vi "Asylum Acquired Data.vi"() -> ()   [LabVIEW 2016]
uses:
  <vilib>/Platform/TimedLoop/XDataNode/timing_clust.ctl
  <vilib>/Platform/TimedLoop/XDataNode/nitl_modes.ctl
  <vilib>/Platform/TimedLoop/XDataNode/wakeup.ctl
  <vilib>/DAQmx/read.llb/DAQmx Read (Analog 1D DBL NChan 1Samp).vi
  subVIs/Driver Variables.vi
  <vilib>/DAQmx/create/channels.llb/DAQmx Create Channel (AI-Voltage-Basic).vi
  <vilib>/DAQmx/configure/timing.llb/DAQmx Timing (Sample Clock).vi
  <vilib>/DAQmx/miscellaneous.llb/DAQmx Fill In Error Info.vi
  <vilib>/Platform/TimedLoop/XDataNode/XDataNode.xnode
  <vilib>/Platform/TimedLoop/XDataNode/XDNodeRunTimeDep.lvlib
panel:
  in  "Reset Graphs":bool
  in  "Data Queue":refnum<queue>
  in  "Skip Back Button":bool
  in  "FF Speed":dbl=2.0
  in  "Progress":dbl(slide)=0.002 scale=0.0..1435.0
  in  "Seek Forward Button":bool
  in  "Media Stop Button":bool
  in  "Play Button":bool
  in  "Tabs":T1(tab)
  in  "Lockin Information":T2={"SR7265 Sensitivity (A)"=5e-07, "Excitation Voltage (V)"=0.1, "SR810 Sensitivity (A)"=0.1, "Femto Gain (V/A)"=1.0, "Frequency (Hz)"=27.0}
  in  "Channel 1 (z, x, y, defl, Vtip, 4t I, 4t V)":tag="Dev1/ai0:3"
  in  "TDMS File Name":string="SA02821"
  in  "TDMS Output Folder":path=path "P:/users1/Yuhe/cypher tdms"
  out "TDMS Path Result":path=path "P:/users1/Yuhe/cypher tdms/SA02821.000109.tdms"
  in  "View Data After?":bool
  out "Z Value":cluster{"Y":dbl[], "Y":dbl[]}[](graph)=[{"Y"=[5.660999774932861, 5.861000061035156, 6.060999870300293, 6.261000156402588, 6.460999965667725, 6.660999774932861, 6.861000061035156, 7.060999870300293, 7.261000156402588, 7.460999965667725, 7.660999774932861, 7.861000061035156, 8.060999870300293, 8.261000156402588, 8.460999965667725, 8.660999774932861, 8.861000061035156, 9.060999870300293, 9.261000156402588, 9.460999965667725, 9.660999774932861, 9.861000061035156, 10.060999870300293, 10.261000156402588, 10.460999965667725, 10.660999774932861, 10.861000061035156, 11.060999870300293, 11.261000156402588, 11.460999965667725, 11.664999961853027, 11.861000061035156, 12.060999870300293, 12.261000156402588, 12.460999965667725, 12.660999774932861, 12.861000061035156, 13.060999870300293, 13.261000156402588, 13.460999965667725, 13.660999774932861, 13.861000061035156, 14.060999870300293, 14.261000156402588, 14.460999965667725, 14.660999774932861, 14.861000061035156, 15.060999870300293, 15.261000156402588, 15.460999965667725, 15.660999774932861, 15.861000061035156, 16.060999870300293, 16.261000156402588, 16.460999965667725, 16.65999984741211, 16.860000133514404, 17.05999994277954, 17.260000228881836, 17.460000038146973, 17.65999984741211, 17.860000133514404, 18.05999994277954, 18.260000228881836, 18.460000038146973, 18.65999984741211, 18.860000133514404, 19.05999994277954, 19.260000228881836, 19.460000038146973, 19.65999984741211, 19.860000133514404, 20.05999994277954, 20.260000228881836, 20.460000038146973, 20.65999984741211, 20.860000133514404, 21.05999994277954, 21.260000228881836, 21.460000038146973, 21.65999984741211, 21.860000133514404, 22.05999994277954, 22.260000228881836, 22.460000038146973, 22.65999984741211, 22.86299991607666, 23.05999994277954, 23.260000228881836, 23.460000038146973, 23.65999984741211, 23.860000133514404, 24.05999994277954, 24.260000228881836, 24.461999893188477, 24.65999984741211, 24.860000133514404, 25.05999994277954, 25.260000228881836, 25.460000038146973, 25.65999984741211, 25.860000133514404, 26.05999994277954, 26.260000228881836, 26.460000038146973], "Y"=[-4.029889960155487, -4.029913362326622, -4.030140697703361, -4.029893303322791, -4.0299033328247065, -4.029686026949883, -4.029659281611442, -4.029562329759599, -4.029849842147827, -4.028997334485054, -4.029719458622933, -4.029826439976692, -4.029873244318962, -4.029833126311303, -4.0292781605386745, -4.029712772288322, -4.029849842147827, -4.029976882505417, -4.0298230968093876, -4.0300303731822975, -4.029535584421158, -4.029806380972862, -4.029916705493927, -4.029910019159317, -4.028963902812004, -4.029986912007331, -4.029776292467117, -4.029923391828537, -4.029960166668892, -4.0288268329524985, -4.030164099874496, -4.029866557984352, -4.030020343680382, -4.029853185315133, -4.029719458622933, -4.029712772288322, -4.029742860794068, -4.029692713284493, -4.030067148022652, -4.029077570500373, -4.030050432186126, -4.029896646490098, -4.029970196170807, -4.029916705493927, -4.029167836017609, -4.029866557984352, -4.0296425657749175, -4.029839812645912, -4.029652595276832, -4.029956823501586, -4.029722801790237, -4.029943450832366, -4.029913362326622, -4.029873244318962, -4.029030766158105, -4.029893303322791, -4.0297328312921525, -4.029809724140167, -4.029502152748108, -4.0292781605386745, -4.029849842147827, -4.0298632148170475, -4.030134011368751, -4.029829783143997, -4.0288268329524985, -4.029776292467117, -4.029933421330452, -4.029525554919243, -4.0298230968093876, -4.0287867149448395, -4.029846498980523, -4.0294754074096675, -4.0296693111133575, -4.029652595276832, -4.028890353131294, -4.029762919797897, -4.029645908942223, -4.029866557984352, -4.029889960155487, -4.028582781739235, -4.029585731930733, -4.029776292467117, -4.029689370117188, -4.029826439976692, -4.029953480334282, -4.029696056451798, -4.030077177524567, -4.029809724140167, -4.0295656729269025, -4.0288769804620745, -4.0299668530035015, -4.029803037805558, -4.030190845212937, -4.029652595276832, -4.030087207026482, -4.029769606132508, -4.029635879440308, -4.029813067307472, -4.029910019159317, -4.029094286336899, -4.0297328312921525, -4.029488780078888, -4.029956823501586, -4.029853185315133, -4.029087600002288]}]
  out "X Position":cluster{"Y":dbl[], "Y":dbl[]}[](graph)=[{"Y"=[5.660999774932861, 5.861000061035156, 6.060999870300293, 6.261000156402588, 6.460999965667725, 6.660999774932861, 6.861000061035156, 7.060999870300293, 7.261000156402588, 7.460999965667725, 7.660999774932861, 7.861000061035156, 8.060999870300293, 8.261000156402588, 8.460999965667725, 8.660999774932861, 8.861000061035156, 9.060999870300293, 9.261000156402588, 9.460999965667725, 9.660999774932861, 9.861000061035156, 10.060999870300293, 10.261000156402588, 10.460999965667725, 10.660999774932861, 10.861000061035156, 11.060999870300293, 11.261000156402588, 11.460999965667725, 11.664999961853027, 11.861000061035156, 12.060999870300293, 12.261000156402588, 12.460999965667725, 12.660999774932861, 12.861000061035156, 13.060999870300293, 13.261000156402588, 13.460999965667725, 13.660999774932861, 13.861000061035156, 14.060999870300293, 14.261000156402588, 14.460999965667725, 14.660999774932861, 14.861000061035156, 15.060999870300293, 15.261000156402588, 15.460999965667725, 15.660999774932861, 15.861000061035156, 16.060999870300293, 16.261000156402588, 16.460999965667725, 16.65999984741211, 16.860000133514404, 17.05999994277954, 17.260000228881836, 17.460000038146973, 17.65999984741211, 17.860000133514404, 18.05999994277954, 18.260000228881836, 18.460000038146973, 18.65999984741211, 18.860000133514404, 19.05999994277954, 19.260000228881836, 19.460000038146973, 19.65999984741211, 19.860000133514404, 20.05999994277954, 20.260000228881836, 20.460000038146973, 20.65999984741211, 20.860000133514404, 21.05999994277954, 21.260000228881836, 21.460000038146973, 21.65999984741211, 21.860000133514404, 22.05999994277954, 22.260000228881836, 22.460000038146973, 22.65999984741211, 22.86299991607666, 23.05999994277954, 23.260000228881836, 23.460000038146973, 23.65999984741211, 23.860000133514404, 24.05999994277954, 24.260000228881836, 24.461999893188477, 24.65999984741211, 24.860000133514404, 25.05999994277954, 25.260000228881836, 25.460000038146973, 25.65999984741211, 25.860000133514404, 26.05999994277954, 26.260000228881836, 26.460000038146973], "Y"=[4.567807958678547, 4.578632321776692, 4.575999827613178, 4.570083792342488, 4.572387932395284, 4.567892877845113, 4.5784454996102495, 4.576243262557331, 4.568481650733296, 4.572693641394917, 4.567853248900715, 4.578802160109822, 4.577307582778279, 4.567428653067891, 4.572982366561238, 4.566811573790853, 4.578666289443317, 4.575846973113362, 4.568175941733663, 4.573129559783284, 4.568815666121785, 4.576679180945699, 4.576107391890828, 4.57247851283962, 4.572659673728292, 4.568532602233234, 4.578541741332355, 4.576724471167866, 4.570383840064351, 4.572263384284321, 4.566709670790974, 4.577443453444783, 4.576639552001301, 4.5702026791756785, 4.572925753783528, 4.567151250457113, 4.578371902999226, 4.577109438056294, 4.572778560561482, 4.573180511283223, 4.569381793898884, 4.5792154333871045, 4.576826374167744, 4.570389501342122, 4.573180511283223, 4.568685456733052, 4.578405870665852, 4.576752777556721, 4.571125467452352, 4.573288075560871, 4.5689005852883495, 4.579113530387227, 4.577183034667317, 4.568487312011068, 4.57270496395046, 4.570916000174824, 4.578932369498554, 4.576464052390401, 4.568651489066426, 4.573214478949848, 4.568742069510762, 4.578654966887775, 4.576849019278828, 4.570797113341634, 4.572552109450641, 4.569495019454305, 4.579034272498433, 4.574612814559284, 4.567281459845845, 4.572801205672566, 4.568793021010701, 4.579124852942769, 4.5765999230569046, 4.5686118601220285, 4.573248446616474, 4.568532602233234, 4.579577755164448, 4.577109438056294, 4.568991165732686, 4.57276723800594, 4.5694440679543655, 4.579441884497944, 4.57680372905666, 4.572059578284565, 4.5720765621178785, 4.569223278121296, 4.575014765281026, 4.576265907668415, 4.567049347457234, 4.572738931617085, 4.565662334403339, 4.579209772109333, 4.577013196334187, 4.574312766837422, 4.572427561339681, 4.569987550620381, 4.578892740554157, 4.5765716166680495, 4.569149681510274, 4.572750254172627, 4.5689062465661205, 4.57850777366573, 4.576135698279683, 4.5765999230569046, 4.572637028617207]}]
  out "Y Position":cluster{"Y":dbl[], "Y":dbl[]}[](graph)=[{"Y"=[5.660999774932861, 5.861000061035156, 6.060999870300293, 6.261000156402588, 6.460999965667725, 6.660999774932861, 6.861000061035156, 7.060999870300293, 7.261000156402588, 7.460999965667725, 7.660999774932861, 7.861000061035156, 8.060999870300293, 8.261000156402588, 8.460999965667725, 8.660999774932861, 8.861000061035156, 9.060999870300293, 9.261000156402588, 9.460999965667725, 9.660999774932861, 9.861000061035156, 10.060999870300293, 10.261000156402588, 10.460999965667725, 10.660999774932861, 10.861000061035156, 11.060999870300293, 11.261000156402588, 11.460999965667725, 11.664999961853027, 11.861000061035156, 12.060999870300293, 12.261000156402588, 12.460999965667725, 12.660999774932861, 12.861000061035156, 13.060999870300293, 13.261000156402588, 13.460999965667725, 13.660999774932861, 13.861000061035156, 14.060999870300293, 14.261000156402588, 14.460999965667725, 14.660999774932861, 14.861000061035156, 15.060999870300293, 15.261000156402588, 15.460999965667725, 15.660999774932861, 15.861000061035156, 16.060999870300293, 16.261000156402588, 16.460999965667725, 16.65999984741211, 16.860000133514404, 17.05999994277954, 17.260000228881836, 17.460000038146973, 17.65999984741211, 17.860000133514404, 18.05999994277954, 18.260000228881836, 18.460000038146973, 18.65999984741211, 18.860000133514404, 19.05999994277954, 19.260000228881836, 19.460000038146973, 19.65999984741211, 19.860000133514404, 20.05999994277954, 20.260000228881836, 20.460000038146973, 20.65999984741211, 20.860000133514404, 21.05999994277954, 21.260000228881836, 21.460000038146973, 21.65999984741211, 21.860000133514404, 22.05999994277954, 22.260000228881836, 22.460000038146973, 22.65999984741211, 22.86299991607666, 23.05999994277954, 23.260000228881836, 23.460000038146973, 23.65999984741211, 23.860000133514404, 24.05999994277954, 24.260000228881836, 24.461999893188477, 24.65999984741211, 24.860000133514404, 25.05999994277954, 25.260000228881836, 25.460000038146973, 25.65999984741211, 25.860000133514404, 26.05999994277954, 26.260000228881836, 26.460000038146973], "Y"=[4.795882738326846, 4.79540291292554, 4.795653730748949, 4.795550132082758, 4.795713708924112, 4.795871833204089, 4.79597543187028, 4.795708256362734, 4.795871833204089, 4.795610110257922, 4.796166271518525, 4.795555584644137, 4.796111745904742, 4.795953621624766, 4.795604657696543, 4.795871833204089, 4.795915453695117, 4.7958118550289255, 4.795708256362734, 4.796068125413713, 4.795642825626193, 4.795631920503434, 4.795582847451029, 4.79593726394063, 4.795839117835818, 4.795997242115793, 4.79554467952138, 4.795740971731005, 4.795959074186144, 4.795708256362734, 4.795795497344789, 4.795501059030352, 4.7962262496936905, 4.79601359979993, 4.796160818957148, 4.795653730748949, 4.796024504922686, 4.795855475519953, 4.795997242115793, 4.795539226960002, 4.795866380642709, 4.795773687099277, 4.795670088433086, 4.7957682345378965, 4.795680993555842, 4.795915453695117, 4.795517416714487, 4.795882738326846, 4.795855475519953, 4.795746424292384, 4.796264417623338, 4.795730066608247, 4.795664635871706, 4.796057220290956, 4.795800949906168, 4.795991789554415, 4.795326577066241, 4.7961008407819845, 4.795392007802781, 4.7956864461172195, 4.795751876853762, 4.795964526747523, 4.796220797132311, 4.7957028038013565, 4.7962262496936905, 4.795882738326846, 4.796035410045442, 4.79589909601098, 4.7961281035888765, 4.795664635871706, 4.7960190523613075, 4.795724614046869, 4.796024504922686, 4.795610110257922, 4.79629713299161, 4.795746424292384, 4.7958118550289255, 4.795877285765467, 4.796073577975092, 4.795670088433086, 4.79589909601098, 4.7961281035888765, 4.795713708924112, 4.796051767729579, 4.79601359979993, 4.795795497344789, 4.795599205135165, 4.795806402467548, 4.795997242115793, 4.795740971731005, 4.7960463151682005, 4.796073577975092, 4.795588300012407, 4.79594271650201, 4.795893643449602, 4.795806402467548, 4.79594271650201, 4.796035410045442, 4.7957682345378965, 4.795833665274438, 4.7962098920095535, 4.7957682345378965, 4.796035410045442, 4.795953621624766, 4.7959699793089]}]
  out "Tip Deflection":cluster{"Y":dbl[], "Y":dbl[]}[](graph)=[{"Y"=[5.660999774932861, 5.861000061035156, 6.060999870300293, 6.261000156402588, 6.460999965667725, 6.660999774932861, 6.861000061035156, 7.060999870300293, 7.261000156402588, 7.460999965667725, 7.660999774932861, 7.861000061035156, 8.060999870300293, 8.261000156402588, 8.460999965667725, 8.660999774932861, 8.861000061035156, 9.060999870300293, 9.261000156402588, 9.460999965667725, 9.660999774932861, 9.861000061035156, 10.060999870300293, 10.261000156402588, 10.460999965667725, 10.660999774932861, 10.861000061035156, 11.060999870300293, 11.261000156402588, 11.460999965667725, 11.664999961853027, 11.861000061035156, 12.060999870300293, 12.261000156402588, 12.460999965667725, 12.660999774932861, 12.861000061035156, 13.060999870300293, 13.261000156402588, 13.460999965667725, 13.660999774932861, 13.861000061035156, 14.060999870300293, 14.261000156402588, 14.460999965667725, 14.660999774932861, 14.861000061035156, 15.060999870300293, 15.261000156402588, 15.460999965667725, 15.660999774932861, 15.861000061035156, 16.060999870300293, 16.261000156402588, 16.460999965667725, 16.65999984741211, 16.860000133514404, 17.05999994277954, 17.260000228881836, 17.460000038146973, 17.65999984741211, 17.860000133514404, 18.05999994277954, 18.260000228881836, 18.460000038146973, 18.65999984741211, 18.860000133514404, 19.05999994277954, 19.260000228881836, 19.460000038146973, 19.65999984741211, 19.860000133514404, 20.05999994277954, 20.260000228881836, 20.460000038146973, 20.65999984741211, 20.860000133514404, 21.05999994277954, 21.260000228881836, 21.460000038146973, 21.65999984741211, 21.860000133514404, 22.05999994277954, 22.260000228881836, 22.460000038146973, 22.65999984741211, 22.86299991607666, 23.05999994277954, 23.260000228881836, 23.460000038146973, 23.65999984741211, 23.860000133514404, 24.05999994277954, 24.260000228881836, 24.461999893188477, 24.65999984741211, 24.860000133514404, 25.05999994277954, 25.260000228881836, 25.460000038146973, 25.65999984741211, 25.860000133514404, 26.05999994277954, 26.260000228881836, 26.460000038146973], "Y"=[2.325611906051636, 2.325635371208191, 2.325648956298828, 2.3255637407302854, 2.3255452156066894, 2.3254772901535032, 2.3255625057220457, 2.3255933809280394, 2.325564975738525, 2.3255476856231687, 2.3256193161010743, 2.325556330680847, 2.325487170219421, 2.325557565689087, 2.325618081092834, 2.3256650114059445, 2.3255736207962037, 2.32559091091156, 2.3255933809280394, 2.325557565689087, 2.3255896759033203, 2.325609436035156, 2.32554274559021, 2.3255921459197997, 2.325582265853882, 2.3255501556396485, 2.325585970878601, 2.325594615936279, 2.3255625057220457, 2.3255748558044433, 2.325567445755005, 2.3255476856231687, 2.325576090812683, 2.325582265853882, 2.3255835008621215, 2.325634136199951, 2.3256193161010743, 2.3255476856231687, 2.325584735870361, 2.325567445755005, 2.3255600357055664, 2.3254772901535032, 2.325599555969238, 2.3255884408950807, 2.325594615936279, 2.325615611076355, 2.3255476856231687, 2.3255056953430175, 2.325584735870361, 2.325571150779724, 2.3255625057220457, 2.325647721290588, 2.3255291604995727, 2.325600790977478, 2.325597085952759, 2.3255538606643675, 2.3254958152770997, 2.325581030845642, 2.325614376068115, 2.325630431175232, 2.3256230211257933, 2.3255143404006957, 2.3254661750793457, 2.325584735870361, 2.3255625057220457, 2.3255341005325314, 2.325551390647888, 2.32554274559021, 2.325603260993957, 2.3255489206314084, 2.32559091091156, 2.325450119972229, 2.3255884408950807, 2.3255835008621215, 2.3255205154418945, 2.325564975738525, 2.3255538606643675, 2.3255686807632445, 2.325537805557251, 2.3256761264801025, 2.3255007553100584, 2.325597085952759, 2.3255872058868405, 2.3256044960021973, 2.325522985458374, 2.3255439805984497, 2.3255588006973267, 2.325556330680847, 2.3255291604995727, 2.3255884408950807, 2.325504460334778, 2.3256254911422727, 2.325584735870361, 2.325489640235901, 2.325582265853882, 2.3255390405654905, 2.325552625656128, 2.3255785608291624, 2.3256366062164306, 2.325620551109314, 2.3256650114059445, 2.32544517993927, 2.325584735870361, 2.3255242204666136, 2.325658836364746]}]
  out "Tip Voltage":cluster{"Y":dbl[], "Y":dbl[]}[](graph)=[{"Y"=[5.660999774932861, 5.861000061035156, 6.060999870300293, 6.261000156402588, 6.460999965667725, 6.660999774932861, 6.861000061035156, 7.060999870300293, 7.261000156402588, 7.460999965667725, 7.660999774932861, 7.861000061035156, 8.060999870300293, 8.261000156402588, 8.460999965667725, 8.660999774932861, 8.861000061035156, 9.060999870300293, 9.261000156402588, 9.460999965667725, 9.660999774932861, 9.861000061035156, 10.060999870300293, 10.261000156402588, 10.460999965667725, 10.660999774932861, 10.861000061035156, 11.060999870300293, 11.261000156402588, 11.460999965667725, 11.664999961853027, 11.861000061035156, 12.060999870300293, 12.261000156402588, 12.460999965667725, 12.660999774932861, 12.861000061035156, 13.060999870300293, 13.261000156402588, 13.460999965667725, 13.660999774932861, 13.861000061035156, 14.060999870300293, 14.261000156402588, 14.460999965667725, 14.660999774932861, 14.861000061035156, 15.060999870300293, 15.261000156402588, 15.460999965667725, 15.660999774932861, 15.861000061035156, 16.060999870300293, 16.261000156402588, 16.460999965667725, 16.65999984741211, 16.860000133514404, 17.05999994277954, 17.260000228881836, 17.460000038146973, 17.65999984741211, 17.860000133514404, 18.05999994277954, 18.260000228881836, 18.460000038146973, 18.65999984741211, 18.860000133514404, 19.05999994277954, 19.260000228881836, 19.460000038146973, 19.65999984741211, 19.860000133514404, 20.05999994277954, 20.260000228881836, 20.460000038146973, 20.65999984741211, 20.860000133514404, 21.05999994277954, 21.260000228881836, 21.460000038146973, 21.65999984741211, 21.860000133514404, 22.05999994277954, 22.260000228881836, 22.460000038146973, 22.65999984741211, 22.86299991607666, 23.05999994277954, 23.260000228881836, 23.460000038146973, 23.65999984741211, 23.860000133514404, 24.05999994277954, 24.260000228881836, 24.461999893188477, 24.65999984741211, 24.860000133514404, 25.05999994277954, 25.260000228881836, 25.460000038146973, 25.65999984741211, 25.860000133514404, 26.05999994277954, 26.260000228881836, 26.460000038146973], "Y"=[0.0, 0.0, 0.0, 0.0, 0.0, 0.0, 0.0, 0.0, 0.0, 0.0, 0.0, 0.0, 0.0, 0.0, 0.0, 0.0, 0.0, 0.0, 0.0, 0.0, 0.0, 0.0, 0.0, 0.0, 0.0, 0.0, 0.0, 0.0, 0.0, 0.0, 0.0, 0.0, 0.0, 0.0, 0.0, 0.0, 0.0, 0.0, 0.0, 0.0, 0.0, 0.0, 0.0, 0.0, 0.0, 0.0, 0.0, 0.0, 0.0, 0.0, 0.0, 0.0, 0.0, 0.0, 0.0, 0.0, 0.0, 0.0, 0.0, 0.0, 0.0, 0.0, 0.0, 0.0, 0.0, 0.0, 0.0, 0.0, 0.0, 0.0, 0.0, 0.0, 0.0, 0.0, 0.0, 0.0, 0.0, 0.0, 0.0, 0.0, 0.0, 0.0, 0.0, 0.0, 0.0, 0.0, 0.0, 0.0, 0.0, 0.0, 0.0, 0.0, 0.0, 0.0, 0.0, 0.0, 0.0, 0.0, 0.0, 0.0, 0.0, 0.0, 0.0, 0.0, 0.0]}]
  out "2-Terminal Conductance":cluster{"Y":dbl[], "Y":dbl[]}[](graph)=[{"Y"=[5.660999774932861, 5.861000061035156, 6.060999870300293, 6.261000156402588, 6.460999965667725, 6.660999774932861, 6.861000061035156, 7.060999870300293, 7.261000156402588, 7.460999965667725, 7.660999774932861, 7.861000061035156, 8.060999870300293, 8.261000156402588, 8.460999965667725, 8.660999774932861, 8.861000061035156, 9.060999870300293, 9.261000156402588, 9.460999965667725, 9.660999774932861, 9.861000061035156, 10.060999870300293, 10.261000156402588, 10.460999965667725, 10.660999774932861, 10.861000061035156, 11.060999870300293, 11.261000156402588, 11.460999965667725, 11.664999961853027, 11.861000061035156, 12.060999870300293, 12.261000156402588, 12.460999965667725, 12.660999774932861, 12.861000061035156, 13.060999870300293, 13.261000156402588, 13.460999965667725, 13.660999774932861, 13.861000061035156, 14.060999870300293, 14.261000156402588, 14.460999965667725, 14.660999774932861, 14.861000061035156, 15.060999870300293, 15.261000156402588, 15.460999965667725, 15.660999774932861, 15.861000061035156, 16.060999870300293, 16.261000156402588, 16.460999965667725, 16.65999984741211, 16.860000133514404, 17.05999994277954, 17.260000228881836, 17.460000038146973, 17.65999984741211, 17.860000133514404, 18.05999994277954, 18.260000228881836, 18.460000038146973, 18.65999984741211, 18.860000133514404, 19.05999994277954, 19.260000228881836, 19.460000038146973, 19.65999984741211, 19.860000133514404, 20.05999994277954, 20.260000228881836, 20.460000038146973, 20.65999984741211, 20.860000133514404, 21.05999994277954, 21.260000228881836, 21.460000038146973, 21.65999984741211, 21.860000133514404, 22.05999994277954, 22.260000228881836, 22.460000038146973, 22.65999984741211, 22.86299991607666, 23.05999994277954, 23.260000228881836, 23.460000038146973, 23.65999984741211, 23.860000133514404, 24.05999994277954, 24.260000228881836, 24.461999893188477, 24.65999984741211, 24.860000133514404, 25.05999994277954, 25.260000228881836, 25.460000038146973, 25.65999984741211, 25.860000133514404, 26.05999994277954, 26.260000228881836, 26.460000038146973], "Y"=[19293.545722961426, 19765.812873840332, 19650.957107543945, 19392.84038543701, 19493.370056152344, 19297.250747680664, 19757.661819458, 19661.57817840576, 19322.938919067383, 19506.708145141598, 19295.52173614502, 19773.22292327881, 19708.014488220215, 19276.996612548828, 19519.30522918701, 19250.073432922363, 19767.294883728027, 19644.288063049316, 19309.600830078125, 19525.72727203369, 19337.512016296387, 19680.597305297848, 19655.65013885498, 19497.32208251953, 19505.226135253906, 19325.161933898926, 19761.86084747314, 19682.573318481445, 19405.93147277832, 19487.93601989746, 19245.627403259277, 19713.942527770996, 19678.868293762203, 19398.027420043945, 19516.83521270752, 19264.893531799316, 19754.450798034664, 19699.369430541992, 19510.41316986084, 19527.950286865234, 19362.212181091305, 19791.2540435791, 19687.01934814453, 19406.17847442627, 19527.950286865234, 19331.830978393555, 19755.932807922367, 19683.80832672119, 19438.288688659668, 19532.64331817627, 19341.21704101562, 19786.80801391602, 19702.580451965332, 19323.185920715332, 19507.2021484375, 19429.149627685547, 19778.903961181644, 19671.21124267578, 19330.34896850586, 19529.43229675293, 19334.300994873047, 19766.800880432125, 19688.007354736324, 19423.96259307861, 19500.53310394287, 19367.152214050293, 19783.349990844727, 19590.441703796387, 19270.57456970215, 19511.401176452637, 19336.52400970459, 19787.30201721191, 19677.139282226562, 19328.619956970215, 19530.914306640625, 19325.161933898926, 19807.062149047848, 19699.369430541992, 19345.169067382812, 19509.91916656494, 19364.92919921875, 19801.13410949707, 19686.031341552734, 19479.04396057129, 19479.784965515133, 19355.29613494873, 19607.97882080078, 19662.566184997555, 19260.44750213623, 19508.68415832519, 19199.93209838867, 19791.007041931152, 19695.170402526855, 19577.350616455078, 19495.09906768799, 19388.641357421875, 19777.174949645996, 19675.904273986816, 19352.08511352539, 19509.178161621094, 19341.464042663574, 19760.37883758545, 19656.885147094727, 19677.139282226562, 19504.23812866211]}]
  out "2-Terminal Resistance":cluster{"Y":dbl[], "Y":dbl[]}[](graph)=[{"Y"=[5.660999774932861, 5.861000061035156, 6.060999870300293, 6.261000156402588, 6.460999965667725, 6.660999774932861, 6.861000061035156, 7.060999870300293, 7.261000156402588, 7.460999965667725, 7.660999774932861, 7.861000061035156, 8.060999870300293, 8.261000156402588, 8.460999965667725, 8.660999774932861, 8.861000061035156, 9.060999870300293, 9.261000156402588, 9.460999965667725, 9.660999774932861, 9.861000061035156, 10.060999870300293, 10.261000156402588, 10.460999965667725, 10.660999774932861, 10.861000061035156, 11.060999870300293, 11.261000156402588, 11.460999965667725, 11.664999961853027, 11.861000061035156, 12.060999870300293, 12.261000156402588, 12.460999965667725, 12.660999774932861, 12.861000061035156, 13.060999870300293, 13.261000156402588, 13.460999965667725, 13.660999774932861, 13.861000061035156, 14.060999870300293, 14.261000156402588, 14.460999965667725, 14.660999774932861, 14.861000061035156, 15.060999870300293, 15.261000156402588, 15.460999965667725, 15.660999774932861, 15.861000061035156, 16.060999870300293, 16.261000156402588, 16.460999965667725, 16.65999984741211, 16.860000133514404, 17.05999994277954, 17.260000228881836, 17.460000038146973, 17.65999984741211, 17.860000133514404, 18.05999994277954, 18.260000228881836, 18.460000038146973, 18.65999984741211, 18.860000133514404, 19.05999994277954, 19.260000228881836, 19.460000038146973, 19.65999984741211, 19.860000133514404, 20.05999994277954, 20.260000228881836, 20.460000038146973, 20.65999984741211, 20.860000133514404, 21.05999994277954, 21.260000228881836, 21.460000038146973, 21.65999984741211, 21.860000133514404, 22.05999994277954, 22.260000228881836, 22.460000038146973, 22.65999984741211, 22.86299991607666, 23.05999994277954, 23.260000228881836, 23.460000038146973, 23.65999984741211, 23.860000133514404, 24.05999994277954, 24.260000228881836, 24.461999893188477, 24.65999984741211, 24.860000133514404, 25.05999994277954, 25.260000228881836, 25.460000038146973, 25.65999984741211, 25.860000133514404, 26.05999994277954, 26.260000228881836, 26.460000038146973], "Y"=[5.1830804682515706e-05, 5.059240449065874e-05, 5.088810659589211e-05, 5.156542209004859e-05, 5.1299492961935945e-05, 5.182085329539442e-05, 5.061327646650814e-05, 5.086061713491017e-05, 5.175196196543506e-05, 5.126441594139825e-05, 5.182549680047088e-05, 5.057344489970375e-05, 5.0740778610535094e-05, 5.1875300914304556e-05, 5.1231331661575256e-05, 5.1947853782716166e-05, 5.058861143530451e-05, 5.090538261251568e-05, 5.178770958549919e-05, 5.121448159486894e-05, 5.1712960755099496e-05, 5.081146595742846e-05, 5.087595642655522e-05, 5.1289094767355635e-05, 5.126831101909615e-05, 5.174600882623736e-05, 5.0602522086267265e-05, 5.080636478874563e-05, 5.153063646559561e-05, 5.13137973656618e-05, 5.1959854518987954e-05, 5.0725520711613205e-05, 5.081593032039243e-05, 5.1551633490666264e-05, 5.123781540917528e-05, 5.190789133349554e-05, 5.062150348920296e-05, 5.076304617393466e-05, 5.125468083601495e-05, 5.1208651461623885e-05, 5.16469910900252e-05, 5.0527369200459084e-05, 5.0794890903291984e-05, 5.152998058416364e-05, 5.1208651461623885e-05, 5.1728157623437824e-05, 5.0617706069489564e-05, 5.0803177078415185e-05, 5.1444857930492705e-05, 5.119634776054306e-05, 5.170305456370026e-05, 5.053872253153223e-05, 5.0754773083555663e-05, 5.1751300437882485e-05, 5.126311771368498e-05, 5.1469056503381446e-05, 5.055891883405744e-05, 5.083571050421879e-05, 5.173212349292084e-05, 5.12047654435027e-05, 5.172154919203823e-05, 5.0589875723893005e-05, 5.0792341854719545e-05, 5.148280095825208e-05, 5.1280649337622826e-05, 5.1633817349487746e-05, 5.054755642814673e-05, 5.1045301332139555e-05, 5.1892588691788876e-05, 5.125208543232925e-05, 5.171560304727578e-05, 5.053746079835208e-05, 5.082039546791505e-05, 5.173675110929913e-05, 5.120088001512526e-05, 5.174600882623736e-05, 5.0487043079635684e-05, 5.076304617393466e-05, 5.169249214193034e-05, 5.1255978636433646e-05, 5.163974470096919e-05, 5.050215782945369e-05, 5.079744020772879e-05, 5.1337221786868005e-05, 5.1335268934964625e-05, 5.1665445624175094e-05, 5.099964708953926e-05, 5.085806148553464e-05, 5.1919873610885064e-05, 5.125922342503337e-05, 5.208351752889396e-05, 5.052799980725098e-05, 5.0773868900961717e-05, 5.107943457678507e-05, 5.129494323306327e-05, 5.157658969318162e-05, 5.056333892712516e-05, 5.082358533945925e-05, 5.1674018284525255e-05, 5.1257925460295563e-05, 5.170239428588193e-05, 5.060631722798446e-05, 5.087275997783399e-05, 5.082039546791505e-05, 5.1270908066409815e-05]}]
  out "4-Terminal Conductance":cluster{"Y":dbl[], "Y":dbl[]}[](graph)=[{"Y"=[5.660999774932861, 5.861000061035156, 6.060999870300293, 6.261000156402588, 6.460999965667725, 6.660999774932861, 6.861000061035156, 7.060999870300293, 7.261000156402588, 7.460999965667725, 7.660999774932861, 7.861000061035156, 8.060999870300293, 8.261000156402588, 8.460999965667725, 8.660999774932861, 8.861000061035156, 9.060999870300293, 9.261000156402588, 9.460999965667725, 9.660999774932861, 9.861000061035156, 10.060999870300293, 10.261000156402588, 10.460999965667725, 10.660999774932861, 10.861000061035156, 11.060999870300293, 11.261000156402588, 11.460999965667725, 11.664999961853027, 11.861000061035156, 12.060999870300293, 12.261000156402588, 12.460999965667725, 12.660999774932861, 12.861000061035156, 13.060999870300293, 13.261000156402588, 13.460999965667725, 13.660999774932861, 13.861000061035156, 14.060999870300293, 14.261000156402588, 14.460999965667725, 14.660999774932861, 14.861000061035156, 15.060999870300293, 15.261000156402588, 15.460999965667725, 15.660999774932861, 15.861000061035156, 16.060999870300293, 16.261000156402588, 16.460999965667725, 16.65999984741211, 16.860000133514404, 17.05999994277954, 17.260000228881836, 17.460000038146973, 17.65999984741211, 17.860000133514404, 18.05999994277954, 18.260000228881836, 18.460000038146973, 18.65999984741211, 18.860000133514404, 19.05999994277954, 19.260000228881836, 19.460000038146973, 19.65999984741211, 19.860000133514404, 20.05999994277954, 20.260000228881836, 20.460000038146973, 20.65999984741211, 20.860000133514404, 21.05999994277954, 21.260000228881836, 21.460000038146973, 21.65999984741211, 21.860000133514404, 22.05999994277954, 22.260000228881836, 22.460000038146973, 22.65999984741211, 22.86299991607666, 23.05999994277954, 23.260000228881836, 23.460000038146973, 23.65999984741211, 23.860000133514404, 24.05999994277954, 24.260000228881836, 24.461999893188477, 24.65999984741211, 24.860000133514404, 25.05999994277954, 25.260000228881836, 25.460000038146973, 25.65999984741211, 25.860000133514404, 26.05999994277954, 26.260000228881836, 26.460000038146973], "Y"=[8.531127129750985, 8.74663897693737, 8.760929413060238, 8.57596941561988, 8.623251748251748, 8.47629380492568, 8.671002710027096, 8.60179381888913, 8.532940663176266, 8.380982701899606, 8.484739871836647, 8.725122615803816, 8.709638685733, 8.508012645808352, 8.461826748045828, 8.46291671191226, 8.729166666666668, 8.710952902519168, 8.519616390584133, 8.673579109062981, 8.452709997840639, 8.678575318592744, 8.69884127678181, 8.62688524590164, 8.37146188911269, 8.572258135203242, 8.70587595212187, 8.712661272687514, 8.600547345374933, 8.327844627401308, 8.58684152523694, 8.710356870020737, 8.73872984534386, 8.567033926039054, 8.582057130444227, 8.46943207731567, 8.69315217391304, 8.654801953336952, 8.677249258486212, 8.411533141823599, 8.606609574000878, 8.75311339305222, 8.727989487516426, 8.588434630520332, 8.435766111822451, 8.541525701189569, 8.665547128927413, 8.689455893577582, 8.528991004660234, 8.655757443082312, 8.505757114925048, 8.764551422319476, 8.718657776806207, 8.539569915948041, 8.390098799532563, 8.592026215182962, 8.701075736172987, 8.675381263616558, 8.440465918895601, 8.466216939715174, 8.537958115183248, 8.732758620689655, 8.775514697787074, 8.571942446043165, 8.333227781296177, 8.531991294885746, 8.760144372744175, 8.560496492174853, 8.502397558849172, 8.327324478178369, 8.538008506925511, 8.632543103448276, 8.638473216222076, 8.480871355803618, 8.362982548915918, 8.509788992821404, 8.68891537544696, 8.703917930808688, 8.55395369156837, 8.273489054153137, 8.478425435276305, 8.723177366702938, 8.648003472222221, 8.595313351498637, 8.631388858487467, 8.504558280876926, 8.723516483516482, 8.671568627450979, 8.427212795849993, 8.349931282376572, 8.511113544289937, 8.72631235025049, 8.795168762409, 8.590007586431126, 8.676156974826867, 8.539599651871193, 8.67298526863085, 8.678396339470531, 8.562622950819671, 8.407919948903556, 8.508638487449744, 8.624514877102198, 8.710814360770579, 8.690302170830153, 8.404001702852279]}]
  out "4-Terminal Resistance":cluster{"Y":dbl[], "Y":dbl[]}[](graph)=[{"Y"=[5.660999774932861, 5.861000061035156, 6.060999870300293, 6.261000156402588, 6.460999965667725, 6.660999774932861, 6.861000061035156, 7.060999870300293, 7.261000156402588, 7.460999965667725, 7.660999774932861, 7.861000061035156, 8.060999870300293, 8.261000156402588, 8.460999965667725, 8.660999774932861, 8.861000061035156, 9.060999870300293, 9.261000156402588, 9.460999965667725, 9.660999774932861, 9.861000061035156, 10.060999870300293, 10.261000156402588, 10.460999965667725, 10.660999774932861, 10.861000061035156, 11.060999870300293, 11.261000156402588, 11.460999965667725, 11.664999961853027, 11.861000061035156, 12.060999870300293, 12.261000156402588, 12.460999965667725, 12.660999774932861, 12.861000061035156, 13.060999870300293, 13.261000156402588, 13.460999965667725, 13.660999774932861, 13.861000061035156, 14.060999870300293, 14.261000156402588, 14.460999965667725, 14.660999774932861, 14.861000061035156, 15.060999870300293, 15.261000156402588, 15.460999965667725, 15.660999774932861, 15.861000061035156, 16.060999870300293, 16.261000156402588, 16.460999965667725, 16.65999984741211, 16.860000133514404, 17.05999994277954, 17.260000228881836, 17.460000038146973, 17.65999984741211, 17.860000133514404, 18.05999994277954, 18.260000228881836, 18.460000038146973, 18.65999984741211, 18.860000133514404, 19.05999994277954, 19.260000228881836, 19.460000038146973, 19.65999984741211, 19.860000133514404, 20.05999994277954, 20.260000228881836, 20.460000038146973, 20.65999984741211, 20.860000133514404, 21.05999994277954, 21.260000228881836, 21.460000038146973, 21.65999984741211, 21.860000133514404, 22.05999994277954, 22.260000228881836, 22.460000038146973, 22.65999984741211, 22.86299991607666, 23.05999994277954, 23.260000228881836, 23.460000038146973, 23.65999984741211, 23.860000133514404, 24.05999994277954, 24.260000228881836, 24.461999893188477, 24.65999984741211, 24.860000133514404, 25.05999994277954, 25.260000228881836, 25.460000038146973, 25.65999984741211, 25.860000133514404, 26.05999994277954, 26.260000228881836, 26.460000038146973], "Y"=[0.11721780680473456, 0.11432963153843495, 0.11414314215607965, 0.11660489481680461, 0.11596553606350302, 0.117976091297885, 0.11532691719451288, 0.11625482227085353, 0.11719289412555853, 0.11931775156929011, 0.11785865293350478, 0.11461157114856552, 0.11481532673905324, 0.11753626297750003, 0.11817779323462502, 0.11816257276981987, 0.11455847386606365, 0.11479800461217107, 0.11737617820948092, 0.11529266049863669, 0.1183052550112318, 0.11522628712805612, 0.11495784089829263, 0.11591669334731647, 0.11945345092544372, 0.1166553778354959, 0.11486495063633045, 0.11477549513055828, 0.11627167103090612, 0.12007909089917274, 0.11645725715406542, 0.11480586001273736, 0.11443310745853154, 0.1167265147197799, 0.11652218069077987, 0.11807167265507022, 0.11503307333146318, 0.1155427954268461, 0.11524389604763347, 0.11888439301466532, 0.1161897728740722, 0.1142450653293554, 0.11457392482973135, 0.11643565500165892, 0.11854288023144935, 0.11707510422502639, 0.11539952373021464, 0.1150820055657691, 0.11724716454482331, 0.1155300409153915, 0.11756743088772703, 0.11409597174169517, 0.11469655502821817, 0.11710191749149398, 0.1191881092001591, 0.11638698330221563, 0.11492831941865893, 0.11526871052004867, 0.11847687336892096, 0.11811651165240442, 0.11712402406075045, 0.11451135372984374, 0.11395343131810988, 0.11665967404244185, 0.12000152140862383, 0.11720593436610915, 0.11415337109359536, 0.11681565579702827, 0.11761388535879541, 0.12008659139308722, 0.11712333278904492, 0.1158407203532666, 0.11576119836758107, 0.11791241369401538, 0.1195745663832678, 0.11751172826902546, 0.11508916456186295, 0.11489079049670775, 0.11690500647393033, 0.12086799239612432, 0.11794642996256459, 0.11463712927365119, 0.11563362743498057, 0.1163424730129114, 0.11585621132134434, 0.117584003628615, 0.11463267288516242, 0.11531939081544126, 0.11866319696575987, 0.11976146607179321, 0.11749344037599391, 0.11459594515097656, 0.11369878604762305, 0.11641433393156075, 0.11525840466317698, 0.11710150972839006, 0.11530055460222396, 0.11522866350027479, 0.11678664556669961, 0.11893548201823141, 0.11752761775315326, 0.11594855198752362, 0.1147998304249846, 0.11507079867299407, 0.11899093399275466]}]
  in  "Background Image":refnum<vi>
  in  "Inkscape File (.svg)":refnum<vi>
  in  "Run":refnum<vi>
  in  "Abort":refnum<vi>
  in  "Lithography Data":T3(array[cluster])=[{"Name"="p0", "Litho"=[{"X"=16.772607, "Y"=18.646625, "Speed"=0.4, "Voltage"=10.0}, {"X"=16.772607, "Y"=18.646625, "Speed"=0.4, "Voltage"=10.0}, {"X"=16.68930094572346, "Y"=18.59130681744784, "Speed"=0.4, "Voltage"=10.0}, {"X"=16.605994891446922, "Y"=18.535988634895677, "Speed"=0.4, "Voltage"=10.0}, {"X"=16.498290179564233, "Y"=18.464468876033056, "Speed"=0.4, "Voltage"=10.0}, {"X"=16.498290179564233, "Y"=18.464468876033056, "Speed"=0.4, "Voltage"=10.0}, {"X"=16.43263695501747, "Y"=18.3890390801523, "Speed"=0.4, "Voltage"=10.0}, {"X"=16.366983730470707, "Y"=18.313609284271546, "Speed"=0.4, "Voltage"=10.0}, {"X"=16.301330505923943, "Y"=18.23817948839079, "Speed"=0.4, "Voltage"=10.0}, {"X"=16.32001038692712, "Y"=18.259641033057846, "Speed"=0.4, "Voltage"=10.0}, {"X"=16.32001038692712, "Y"=18.259641033057846, "Speed"=0.4, "Voltage"=10.0}, {"X"=16.281074071824737, "Y"=18.16753260040237, "Speed"=0.4, "Voltage"=10.0}, {"X"=16.227126534184823, "Y"=18.0399133553719, "Speed"=0.4, "Voltage"=10.0}, {"X"=16.227126534184823, "Y"=18.0399133553719, "Speed"=0.4, "Voltage"=10.0}, {"X"=16.219160503904092, "Y"=17.940231148526514, "Speed"=0.4, "Voltage"=10.0}, {"X"=16.20899753343351, "Y"=17.813057727272724, "Speed"=0.4, "Voltage"=10.0}, {"X"=16.20899753343351, "Y"=17.813057727272724, "Speed"=0.4, "Voltage"=10.0}, {"X"=16.22891830037272, "Y"=17.71506199754661, "Speed"=0.4, "Voltage"=10.0}, {"X"=16.248839067311923, "Y"=17.617066267820494, "Speed"=0.4, "Voltage"=10.0}, {"X"=16.254982296769345, "Y"=17.586846033057846, "Speed"=0.4, "Voltage"=10.0}, {"X"=16.254982296769345, "Y"=17.586846033057846, "Speed"=0.4, "Voltage"=10.0}, {"X"=16.296521515711, "Y"=17.49588179123878, "Speed"=0.4, "Voltage"=10.0}, {"X"=16.33806073465265, "Y"=17.404917549419714, "Speed"=0.4, "Voltage"=10.0}, {"X"=16.354439736288505, "Y"=17.369050157024795, "Speed"=0.4, "Voltage"=10.0}, {"X"=16.354439736288505, "Y"=17.369050157024795, "Speed"=0.4, "Voltage"=10.0}, {"X"=16.412101936590453, "Y"=17.28734905142433, "Speed"=0.4, "Voltage"=10.0}, {"X"=16.469764136892397, "Y"=17.205647945823866, "Speed"=0.4, "Voltage"=10.0}, {"X"=16.49672876408715, "Y"=17.167441983471072, "Speed"=0.4, "Voltage"=10.0}, {"X"=16.49672876408715, "Y"=17.167441983471072, "Speed"=0.4, "Voltage"=10.0}, {"X"=16.5668002273979, "Y"=17.09609781742023, "Speed"=0.4, "Voltage"=10.0}, {"X"=16.636871690708645, "Y"=17.024753651369384, "Speed"=0.4, "Voltage"=10.0}, {"X"=16.671208292261458, "Y"=16.989793396694218, "Speed"=0.4, "Voltage"=10.0}, {"X"=16.671208292261458, "Y"=16.989793396694218, "Speed"=0.4, "Voltage"=10.0}, {"X"=16.751424732113648, "Y"=16.93008307281769, "Speed"=0.4, "Voltage"=10.0}, {"X"=16.83164117196584, "Y"=16.87037274894116, "Speed"=0.4, "Voltage"=10.0}, {"X"=16.86723723290759, "Y"=16.843876280991736, "Speed"=0.4, "Voltage"=10.0}, {"X"=16.86723723290759, "Y"=16.843876280991736, "Speed"=0.4, "Voltage"=10.0}, {"X"=16.956167956471436, "Y"=16.79814525862824, "Speed"=0.4, "Voltage"=10.0}, {"X"=17.045098680035284, "Y"=16.752414236264737, "Speed"=0.4, "Voltage"=10.0}, {"X"=17.074174498121714, "Y"=16.737462520661154, "Speed"=0.4, "Voltage"=10.0}, {"X"=17.074174498121714, "Y"=16.737462520661154, "Speed"=0.4, "Voltage"=10.0}, {"X"=17.17033458342018, "Y"=16.710017339018613, "Speed"=0.4, "Voltage"=10.0}, {"X"=17.266494668718643, "Y"=16.682572157376075, "Speed"=0.4, "Voltage"=10.0}, {"X"=17.281379, "Y"=16.678324, "Speed"=0.4, "Voltage"=10.0}, {"X"=17.281379, "Y"=16.678324, "Speed"=0.4, "Voltage"=10.0}, {"X"=17.381379000000003, "Y"=16.678324, "Speed"=0.4, "Voltage"=10.0}, {"X"=17.481379, "Y"=16.678324, "Speed"=0.4, "Voltage"=10.0}, {"X"=17.581379000000002, "Y"=16.678324, "Speed"=0.4, "Voltage"=10.0}, {"X"=17.681379, "Y"=16.678324, "Speed"=0.4, "Voltage"=10.0}, {"X"=17.781379, "Y"=16.678324, "Speed"=0.4, "Voltage"=10.0}, {"X"=17.781379, "Y"=16.678324, "Speed"=0.4, "Voltage"=10.0}, {"X"=17.781379, "Y"=16.678324, "Speed"=0.4, "Voltage"=10.0}, {"X"=17.88061144583518, "Y"=16.69069015112185, "Speed"=0.4, "Voltage"=10.0}, {"X"=17.979843891670356, "Y"=16.7030563022437, "Speed"=0.4, "Voltage"=10.0}, {"X"=18.079076337505537, "Y"=16.71542245336555, "Speed"=0.4, "Voltage"=10.0}, {"X"=18.178308783340714, "Y"=16.7277886044874, "Speed"=0.4, "Voltage"=10.0}, {"X"=18.266695387678432, "Y"=16.738803168294513, "Speed"=0.4, "Voltage"=10.0}, {"X"=18.266695387678432, "Y"=16.738803168294513, "Speed"=0.4, "Voltage"=10.0}, {"X"=18.36417973848919, "Y"=16.761092209256496, "Speed"=0.4, "Voltage"=10.0}, {"X"=18.46166408929995, "Y"=16.783381250218476, "Speed"=0.4, "Voltage"=10.0}, {"X"=18.559148440110707, "Y"=16.80567029118046, "Speed"=0.4, "Voltage"=10.0}, {"X"=18.649982960931627, "Y"=16.82643890007513, "Speed"=0.4, "Voltage"=10.0}, {"X"=18.649982960931627, "Y"=16.82643890007513, "Speed"=0.4, "Voltage"=10.0}, {"X"=18.743972407715418, "Y"=16.860585406386562, "Speed"=0.4, "Voltage"=10.0}, {"X"=18.837961854499213, "Y"=16.894731912697992, "Speed"=0.4, "Voltage"=10.0}, {"X"=18.931951301283004, "Y"=16.928878419009425, "Speed"=0.4, "Voltage"=10.0}, {"X"=18.948125516904582, "Y"=16.93475453568745, "Speed"=0.4, "Voltage"=10.0}, {"X"=18.948125516904582, "Y"=16.93475453568745, "Speed"=0.4, "Voltage"=10.0}, {"X"=19.03637427659975, "Y"=16.981788102554788, "Speed"=0.4, "Voltage"=10.0}, {"X"=19.124623036294917, "Y"=17.02882166942213, "Speed"=0.4, "Voltage"=10.0}, {"X"=19.1780068527423, "Y"=17.057273415477084, "Speed"=0.4, "Voltage"=10.0}, {"X"=19.1780068527423, "Y"=17.057273415477084, "Speed"=0.4, "Voltage"=10.0}, {"X"=19.25878899612575, "Y"=17.116216144548407, "Speed"=0.4, "Voltage"=10.0}, {"X"=19.339571139509204, "Y"=17.175158873619733, "Speed"=0.4, "Voltage"=10.0}, {"X"=19.35651076558978, "Y"=17.18751887978963, "Speed"=0.4, "Voltage"=10.0}, {"X"=19.35651076558978, "Y"=17.18751887978963, "Speed"=0.4, "Voltage"=10.0}, {"X"=19.430357339713883, "Y"=17.25494797951766, "Speed"=0.4, "Voltage"=10.0}, {"X"=19.50052105259204, "Y"=17.319014268970697, "Speed"=0.4, "Voltage"=10.0}, {"X"=19.50052105259204, "Y"=17.319014268970697, "Speed"=0.4, "Voltage"=10.0}, {"X"=19.571268607048314, "Y"=17.38968805151031, "Speed"=0.4, "Voltage"=10.0}, {"X"=19.626921510894064, "Y"=17.445282923365887, "Speed"=0.4, "Voltage"=10.0}, {"X"=19.626921510894064, "Y"=17.445282923365887, "Speed"=0.4, "Voltage"=10.0}, {"X"=19.700823022644997, "Y"=17.512651807584987, "Speed"=0.4, "Voltage"=10.0}, {"X"=19.752595937640873, "Y"=17.559848183320813, "Speed"=0.4, "Voltage"=10.0}, {"X"=19.752595937640873, "Y"=17.559848183320813, "Speed"=0.4, "Voltage"=10.0}, {"X"=19.83530503946557, "Y"=17.61605498429144, "Speed"=0.4, "Voltage"=10.0}, {"X"=19.894428129977463, "Y"=17.656233389181068, "Speed"=0.4, "Voltage"=10.0}, {"X"=19.894428129977463, "Y"=17.656233389181068, "Speed"=0.4, "Voltage"=10.0}, {"X"=19.986947701576806, "Y"=17.69418241909059, "Speed"=0.4, "Voltage"=10.0}, {"X"=20.069301885048837, "Y"=17.72796188129226, "Speed"=0.4, "Voltage"=10.0}, {"X"=20.069301885048837, "Y"=17.72796188129226, "Speed"=0.4, "Voltage"=10.0}, {"X"=20.167710182029342, "Y"=17.74573284315133, "Speed"=0.4, "Voltage"=10.0}, {"X"=20.266118479009847, "Y"=17.763503805010405, "Speed"=0.4, "Voltage"=10.0}, {"X"=20.294101, "Y"=17.768557, "Speed"=0.4, "Voltage"=10.0}]}, ...(14 in all)]
  # "FUTURE: will be used for TDMS playback"
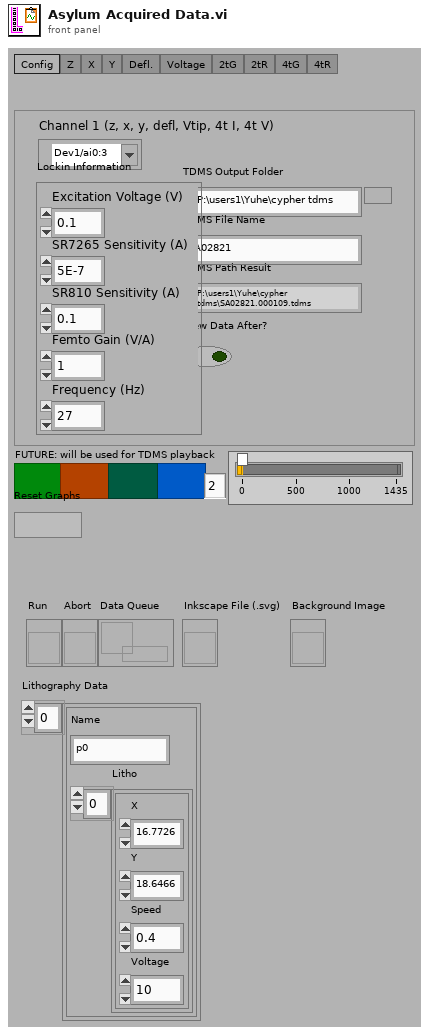
[diagram p1: front panel]
types:
  T1 = enum32{"Config", "Z", "X", "Y", "Defl.", "Voltage", "2tG", "2tR", "4tG", "4tR"}
  T2 = cluster{"SR7265 Sensitivity (A)":dbl, "Excitation Voltage (V)":dbl, "SR810 Sensitivity (A)":dbl, "Femto Gain (V/A)":dbl, "Frequency (Hz)":dbl}
  T3 = cluster{"Name":string, "Litho":cluster{"X":dbl, "Y":dbl, "Speed":dbl, "Voltage":dbl}[]}[]
  T4 = typedef "XDNodeRunTimeDep.lvlib/timing_clust.ctl" = cluster{"Expected End [f-1]":u64, "Actual End [f-1]":u64, "Finished Late? [f-1]":bool, "Expected End [i-1]":u64, "Actual End [i-1]":u64, "Finished Late? [i-1]":bool, "Expected Start [i]":u64, "Actual Start [i]":u64, "Expected Start [f]":u64, "Actual Start [f]":u64, "Source Name":string, "Structure Name":string, "Period":i64, "Deadline":i64, "Offset":i64, "Start":i64, "Priority":i32, "Timeout":i32, "Mode":T5, "Wakeup Reason":T6, "Error":errorcluster, "Source Type":string, "Secondary Source Type":string, "Global End Time":u64, "Global Start Time":u64, "Frame Duration":u64, "Iteration Duration":u64, "Assigned CPU":i32, "I/O Scan Engine Mode":u32}
  T5 = typedef "XDNodeRunTimeDep.lvlib/nitl_modes.ctl" = enum32{"No Change", "Process missed periods, maintain original phase", "Discard missed periods, maintain original phase", "Process missed periods, ignore original phase", "Discard missed periods, ignore original phase"}
  T6 = typedef "XDNodeRunTimeDep.lvlib/wakeup.ctl" = enum32{"Normal", "Aborted", "Asynchronous wakeup", "Timing source error", "Timed loop error", "Timeout"}
  T7 = cluster{"Result":dbl, "Result":dbl, "Result":dbl, "Result":dbl, "Result":dbl, "Result":dbl}
  T8 = cluster{"SR7265 Sensitivity (A)":dbl, "Excitation Voltage (V)":dbl, "Femto Gain (V/A)":dbl, "SR810 Sensitivity (A)":dbl}
  T9 = cluster{"x":dbl, "y":dbl, "Voltage":dbl, "Voltage":dbl}
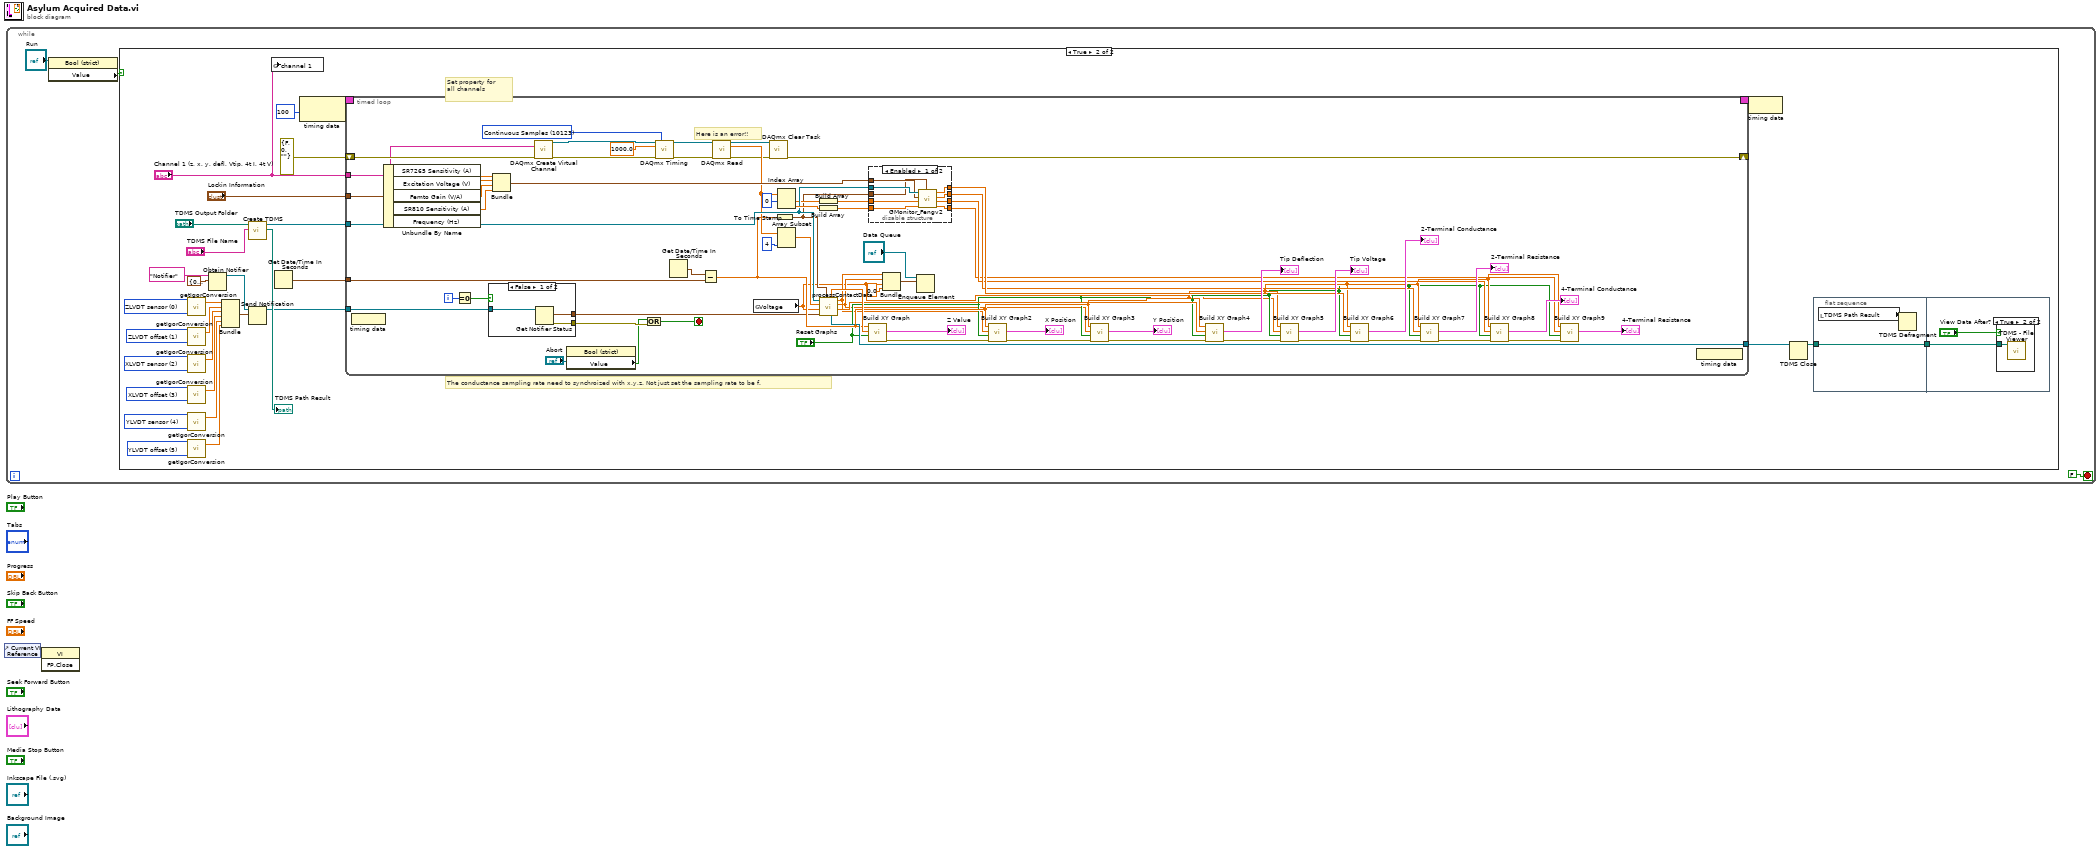
[diagram p0: block diagram]
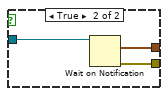
[diagram p5: hidden frame]
diagram:
  n1 = control-ref of="Current VI Reference"() -> (w1:refnum<vi>)
  n2 = while {
    stop <- FALSE stop-if-true
    n3 = property class="Bool (strict)"(reference="Run") -> ("Value"=w3:bool)  [unwired: 1 in, 2 out]
    n4 = case shown="True" w3 {
      frame False {
      }
      frame True {
        w16 = 5 items=["ZLVDT sensor", "ZLVDT offset", "XLVDT sensor", "XLVDT offset", "YLVDT sensor", "YLVDT offset", "DEFL"] ("index")
        w17 = 4 items=["ZLVDT sensor", "ZLVDT offset", "XLVDT sensor", "XLVDT offset", "YLVDT sensor", "YLVDT offset", "DEFL"] ("index")
        w18 = 3 items=["ZLVDT sensor", "ZLVDT offset", "XLVDT sensor", "XLVDT offset", "YLVDT sensor", "YLVDT offset", "DEFL"] ("index")
        w19 = 2 items=["ZLVDT sensor", "ZLVDT offset", "XLVDT sensor", "XLVDT offset", "YLVDT sensor", "YLVDT offset", "DEFL"] ("index")
        w20 = 1 items=["ZLVDT sensor", "ZLVDT offset", "XLVDT sensor", "XLVDT offset", "YLVDT sensor", "YLVDT offset", "DEFL"] ("index")
        w21 = 0 items=["ZLVDT sensor", "ZLVDT offset", "XLVDT sensor", "XLVDT offset", "YLVDT sensor", "YLVDT offset", "DEFL"] ("index")
        # "Set property for \nall channels"
        # "The conductance sampling rate need to synchroized with x,y,z. Not just set the sampling rate to be f."
        n5 = call "getIgorConversion.vi"("index"=w21) -> ("Result"=w15:dbl)  [unwired: 1 out]
        n6 = call "getIgorConversion.vi"("index"=w20) -> ("Result"=w14:dbl)  [unwired: 1 out]
        n7 = call "getIgorConversion.vi"("index"=w19) -> ("Result"=w13:dbl)  [unwired: 1 out]
        n8 = call "getIgorConversion.vi"("index"=w18) -> ("Result"=w12:dbl)  [unwired: 1 out]
        n9 = call "getIgorConversion.vi"("index"=w17) -> ("Result"=w11:dbl)  [unwired: 1 out]
        n10 = call "getIgorConversion.vi"("index"=w16) -> ("Result"=w10:dbl)  [unwired: 1 out]
        n11 = Obtain Notifier(name (unnamed)="Notifier", notification data type=cluster{dbl, dbl, dbl, dbl, dbl, dbl} {0.0, 0.0, 0.0, 0.0, 0.0, 0.0}) -> (notifier out=w8:refnum<notifier>)  [unwired: 2 in, 2 out]
        n12 = Bundle("Result"=w15, "Result"=w14, "Result"=w13, "Result"=w12, "Result"=w11, "Result"=w10) -> (w9:T7)  [unwired: 1 in]
        n13 = call "Create TDMS.vi"("TDMS File Name"="TDMS File Name", "TDMS Output Folder"="TDMS Output Folder") -> ("modified path"=→"TDMS Path Result":path, "Refnum out"=w24:refnum<k34>)  [unwired: 8 in]
        n14 = Send Notification(notification=w9, notifier=w8) -> (notifier out=w6:refnum<notifier>)  [unwired: 1 in, 1 out]
        n15 = global write "Driver Variables.vi" "channel 1"("Channel 1 (z, x, y, defl, Vtip, 4t I, 4t V)") -> ()
        n16 = Get Date/Time In Seconds() -> (seconds since 1Jan1904=w26:timestamp)
        n17 = node-c288(100) -> (w35:T4)
        n18 = timed-loop {
          timing: w35 -> [_]
          timing-out: [_] -> w34
          tunnel: w6 -> [w107]
          tunnel: w24 -> [w102]
          shift-right: [w64] -> _
          shift-left: errorcluster {"status"=FALSE, "code"=0, "source"=""} ("error out") -> [w58]
          tunnel: "Lockin Information" -> [w101]
          tunnel: [w103] -> w28
          tunnel: w26 -> [w95]
          tunnel: "Channel 1 (z, x, y, defl, Vtip, 4t I, 4t V)" -> [w55]
          i -> [w109]
          stop <- w48 stop-if-true
          w62 = 10123 items=["Finite Samples"=10178, "Continuous Samples"=10123, "Hardware Timed Single Point"=12522] ("sample mode")
          # "Here is an error!!"
          n19 = node-c288() -> ()  [unwired: 1 in]
          n20 = Unbundle By Name(w101) -> ("SR7265 Sensitivity (A)"=w96:dbl, "Excitation Voltage (V)"=w100:dbl, "Femto Gain (V/A)"=w99:dbl, "SR810 Sensitivity (A)"=w98:dbl)  [unwired: 1 out]
          n21 = Equal To 0?(x=w109) -> (x = 0?=w108:bool)
          n22 = case shown="False" w108 {
            tunnel: w107 -> [w121 w124]
            tunnel: [w120 w123] -> w50
            tunnel: [w119 w122] -> w52
            frame False {
              n23 = Get Notifier Status(notifier=w121) -> (current notification=w119:cluster{dbl, dbl, dbl, dbl, dbl, dbl}, error out=w120:errorcluster)  [unwired: 1 in, 3 out]
            }
            frame True {
              n24 = Wait on Notification(notifier=w124) -> (notification=w122:cluster{dbl, dbl, dbl, dbl, dbl, dbl}, error out=w123:errorcluster)  [unwired: 3 in, 2 out]
            }
          }
          n25 = Bundle("SR7265 Sensitivity (A)"=w96, "Excitation Voltage (V)"=w100, "Femto Gain (V/A)"=w99, "SR810 Sensitivity (A)"=w98) -> (w97:T8)  [unwired: 1 in]
          n26 = call-poly <vilib>:"DAQmx Create Virtual Channel.vi"("physical channels"=w55, "error in"=w58) -> ("task out"=w61:refnum<k21>, "error out"=w60:errorcluster)  [unwired: 12 in]
          n27 = property class="Bool (strict)"(reference="Abort") -> ("Value"=w49:bool)  [unwired: 1 in, 2 out]
          n28 = Or(x=w49, y=w50) -> (x .or. y?=w48:bool)
          n29 = call-poly <vilib>:"DAQmx Timing.vi"("task/channels in"=w61, "sample mode"=w62, "rate"=1000.0, "error in"=w60) -> ("task out"=w59:refnum<k21>, "error out"=w57:errorcluster)  [unwired: 10 in]
          n30 = Get Date/Time In Seconds() -> (seconds since 1Jan1904=w92:timestamp)
          n31 = Subtract(x=w92, y=w95) -> (x-y=w54:dbl)
          n32 = call-poly <vilib>:"DAQmx Read.vi"("task/channels in"=w59, "error in"=w57) -> ("task out"=w56:refnum<k21>, "data"=w66:dbl[], "error out"=w65:errorcluster)  [unwired: 11 in]
          n33 = global read "Driver Variables.vi" "Voltage"() -> (w44:dbl)
          n34 = call <vilib>:"DAQmx Clear Task.vi"("task in"=w56, "error in"=w65) -> ("error out"=w64:errorcluster)  [unwired: 13 in]
          n35 = To Time Stamp(1:w54) -> (0:w53:timestamp)
          n36 = Index Array(array=w66, index #1=0) -> (element #1=w78:dbl, element #2=w105:dbl)  [unwired: 1 in]
          n37 = Array Subset(array=w66, length=4) -> (w67:dbl[])  [unwired: 1 in]
          n38 = Build Array(w78) -> (w77:dbl[])
          n39 = Build Array(w105) -> (w104:dbl[])
          n40 = call "processContactData.vi"("tdms file"=w102, "data"=w67, "tip voltage"=w44, "lvdt"=w52, "time stamp"=w53) -> ("z"=w93:dbl, "tdms file out"=w103:refnum<k34>, "x"=w46:dbl, "y"=w45:dbl, "deflection"=w88:dbl)  [unwired: 1 out]
          n41 = disable-structure shown="Enabled" {
            disable-tunnel: w104 -> [w118 _]
            disable-tunnel: w102 -> [w117 _]
            disable-tunnel: w97 -> [w116 _]
            disable-tunnel: w53 -> [w115 _]
            disable-tunnel: [w114 _] -> w85
            disable-tunnel: [w113 _] -> w83
            disable-tunnel: [w112 _] -> w80
            disable-tunnel: [w111 _] -> w79
            disable-tunnel: w77 -> [w110 _]
            frame Enabled {
              n42 = call "GMonitor_Fengv2.vi"("Time Stamp"=w115, "v1"=w118, "v0"=w110, "lockin information"=w116, "tdms file"=w117) -> ("FtR"=w111:dbl, "FtG"=w112:dbl, "TtR"=w113:dbl, "TtG"=w114:dbl)  [unwired: 1 out]
            }
            frame Disabled {
            }
          }
          n43 = call "Build XY Graph"("Reset"="Reset Graphs", "Y Input"=w93, "X Input"=w54) -> ("error out"=w76:errorcluster, "XY Graph"=→"Z Value":cluster{"X":dbl[], "Y":dbl[]}[])  [unwired: 7 in]
          n44 = Bundle("x"=w46, "y"=w45, "Voltage"=w44, "Voltage"=0.0) -> (w42:T9)  [unwired: 1 in]
          n45 = Enqueue Element(queue="Data Queue", element=w42) -> ()  [unwired: 2 in, 3 out]
          n46 = call "Build XY Graph2"("error in (no error)"=w76, "Reset"="Reset Graphs", "Y Input"=w46, "X Input"=w54) -> ("error out"=w75:errorcluster, "XY Graph"=→"X Position":cluster{"X":dbl[], "Y":dbl[]}[])  [unwired: 6 in]
          n47 = call "Build XY Graph3"("error in (no error)"=w75, "Reset"="Reset Graphs", "Y Input"=w45, "X Input"=w54) -> ("error out"=w74:errorcluster, "XY Graph"=→"Y Position":cluster{"X":dbl[], "Y":dbl[]}[])  [unwired: 6 in]
          n48 = call "Build XY Graph4"("error in (no error)"=w74, "Reset"="Reset Graphs", "Y Input"=w88, "X Input"=w54) -> ("error out"=w73:errorcluster, "XY Graph"=→"Tip Deflection":cluster{"X":dbl[], "Y":dbl[]}[])  [unwired: 6 in]
          n49 = call "Build XY Graph5"("error in (no error)"=w73, "Reset"="Reset Graphs", "Y Input"=w44, "X Input"=w54) -> ("error out"=w72:errorcluster, "XY Graph"=→"Tip Voltage":cluster{"X":dbl[], "Y":dbl[]}[])  [unwired: 6 in]
          n50 = call "Build XY Graph6"("error in (no error)"=w72, "Reset"="Reset Graphs", "Y Input"=w85, "X Input"=w54) -> ("error out"=w71:errorcluster, "XY Graph"=→"2-Terminal Conductance":cluster{"X":dbl[], "Y":dbl[]}[])  [unwired: 6 in]
          n51 = call "Build XY Graph7"("error in (no error)"=w71, "Reset"="Reset Graphs", "Y Input"=w83, "X Input"=w54) -> ("error out"=w70:errorcluster, "XY Graph"=→"2-Terminal Resistance":cluster{"X":dbl[], "Y":dbl[]}[])  [unwired: 6 in]
          n52 = call "Build XY Graph8"("error in (no error)"=w70, "Reset"="Reset Graphs", "Y Input"=w80, "X Input"=w54) -> ("error out"=w69:errorcluster, "XY Graph"=→"4-Terminal Conductance":cluster{"X":dbl[], "Y":dbl[]}[])  [unwired: 6 in]
          n53 = call "Build XY Graph9"("error in (no error)"=w69, "Reset"="Reset Graphs", "Y Input"=w79, "X Input"=w54) -> ("XY Graph"=→"4-Terminal Resistance":cluster{"X":dbl[], "Y":dbl[]}[])  [unwired: 6 in, 1 out]
          n54 = node-c288() -> ()  [unwired: 1 out]
        }
        n55 = node-c288(w34) -> ()
        n56 = TDMS Close(11:w28) -> (3:w27:path)  [unwired: 1 in, 1 out]
        n57 = flat-sequence {
          tunnel: w27 -> [w37]
          tunnel: [w37] -> w33
          tunnel: w33 -> [w39]
          frame #0 {
            n58 = local read "TDMS Path Result"() -> (w36:path)
            n59 = TDMS Defragment(7:w36) -> ()  [unwired: 1 in, 1 out]
          }
          frame #1 {
            n60 = case shown="True" "View Data After?" {
              tunnel: w39 -> [_ w40]
              frame False {
              }
              frame True {
                n61 = call <vilib>:"TDMS - File Viewer.vi"("file path"=w40) -> ()  [unwired: 5 in, 2 out]
              }
            }
          }
        }
      }
    }
  }
  n62 = invoke class="VI" method="FP.Close"(reference=w1) -> ()  [unwired: 2 in, 3 out]
